vi "CMD - show panel.vi"(8 "error in (no error)":errorcluster, 10 "TipPanel":refnum<class "TipPanel.lvclass">, 11 "TipPanelHandle":refnum<class "TipPanelHandle.lvclass">) -> (0 "error out":errorcluster, 3 "TipPanelHandle":refnum<class "TipPanelHandle.lvclass">)   [LabVIEW 2021, in "TipStripOOPanel.lvlib" / "TipPanelHandle.lvclass"]
uses:
  TipPanelHandle.lvclass
  TipPanel/TipPanel.lvclass
  SubVIs/tipstrip UE data.ctl
  SubVIs/tipstrip action.ctl
  TipPanelHandle.lvclass/TipPanelHandle.ctl
  TipStripOOPanel.lvlib
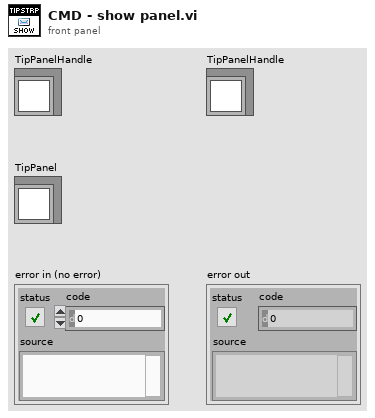
[diagram p1: front panel]
types:
  T1 = typedef "TipStripOOPanel.lvlib/tipstrip action.ctl" = enum16{"hide", "show"}
  T2 = typedef "TipStripOOPanel.lvlib/tipstrip UE data.ctl" = cluster{"action":T1, "TipPanel":refnum<class "TipPanel.lvclass">}
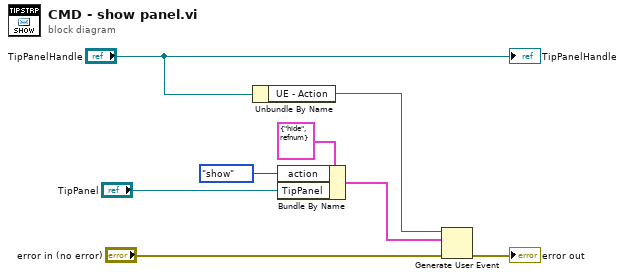
[diagram p0: block diagram]
diagram:
  n1 = Unbundle By Name("TipPanelHandle") -> ("UE - Action"=w5:refnum<user-event>)
  n2 = Bundle By Name(cluster=T2 {"action"=enum."hide", "TipPanel"=refnum} ("Data"), "action"=tipstrip_action."show", "TipPanel"="TipPanel") -> (w4:T2)
  n3 = Generate User Event(user event=w5, event data cluster=w4, error in="error in (no error)") -> (error out=→"error out":errorcluster)  [unwired: 1 in, 1 out]
  "TipPanelHandle" <- "TipPanelHandle"
